vi "Calculate Center.vi"(11 "Rectangle":T1) -> (3 "Center":cluster{"x":i32, "y":i32})   [LabVIEW 2012]
doc: "Calculates the center of a rectangle"
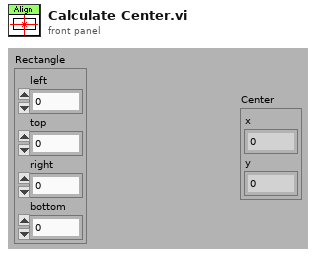
[diagram p1: front panel]
types:
  T1 = cluster{"left":i16, "top":i16, "right":i16, "bottom":i16}
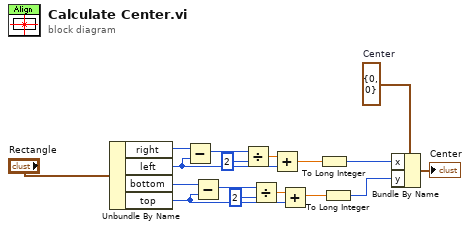
[diagram p0: block diagram]
diagram:
  w6 = cluster{"x":i32, "y":i32} {"x"=0, "y"=0}  # Center
  n1 = Unbundle By Name("Rectangle") -> ("right"=w14:i16, "left"=w12:i16, "bottom"=w8:i16, "top"=w7:i16)
  n2 = Subtract(x=w14, y=w12) -> (x-y=w13:i16)
  n3 = Subtract(x=w8, y=w7) -> (x-y=w11:i16)
  n4 = Divide(x=w13, y=i16 2) -> (x/y=w15:dbl)
  n5 = Divide(x=w11, y=i16 2) -> (x/y=w10:dbl)
  n6 = Add(x=w15, y=w12) -> (x+y=w5:dbl)
  n7 = Add(x=w10, y=w7) -> (x+y=w4:dbl)
  n8 = To Long Integer(number=w5) -> (32bit integer=w3:i32)
  n9 = To Long Integer(number=w4) -> (32bit integer=w2:i32)
  n10 = Bundle By Name(cluster=w6, "x"=w3, "y"=w2) -> (→"Center":cluster{"x":i32, "y":i32})
